vi "AddVertex.vi"(9 "DAG in":refnum<class "DAG.lvclass">) -> (3 "DAG out":refnum<class "DAG.lvclass">, 4 "vertex out":i32)   [LabVIEW 2014, in "DAG.lvclass"]
uses:
  DAG.lvclass
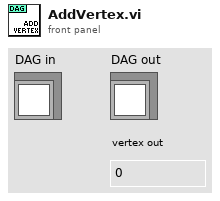
[diagram p1: front panel]
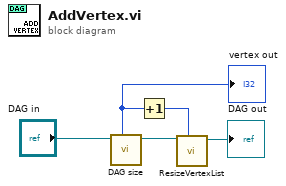
[diagram p0: block diagram]
diagram:
  n1 = call "DAG size.vi"("DAG in"="DAG in") -> ("DAG out"=w4:refnum<class "DAG.lvclass">, "vertices"=w1:i32)  [unwired: 6 in, 1 out]
  "vertex out" <- w1
  n2 = Increment(x=w1) -> (x+1=w3:i32)
  n3 = call "ResizeVertexList.vi"("size"=w3, "DAG in"=w4) -> ("DAG out"=→"DAG out":refnum<class "DAG.lvclass">)  [unwired: 7 in]
